vi "Panel.vi"(11 "LightsPanel in":refnum<class "LightsPanel.lvclass">) -> ()   [LabVIEW 2022 SP3, in "TouchControl.lvlib" / "LightsPanel.lvclass"]
uses:
  LightsPanel.lvclass
  C:/Program Files (x86)/National Instruments/LabVIEW 2022/vi.lib/IlluminatedG/IG OOPanel/OOPanel/Panel/Panel.lvclass
  Temperature Meter.ctl
  <vilib>/IlluminatedG/IG OOPanel/OOPanel/Panel/Basic UI State.ctl
  Light Selection.ctl
  <vilib>/IlluminatedG/IG OOPanel/OOPanel/Panel/Panel.lvclass
  <vilib>/IlluminatedG/IG OOPanel/OOPanel/OOPanel.lvlib
  TouchControl.lvlib
panel:
  in  "Printer On":bool
  in  "Desk Right On":bool
  in  "Desk Left On":bool
  in  "Printer Brightness":i32(slide) caption="Printer" scale=3.0..100.0
  in  "Printer Temp":T1 scale=7000.0..2900.0
  in  "Link":bool=TRUE
  in  "Desk Right Temp":T1 scale=7000.0..2900.0
  in  "Desk Right Brightness":i32(slide) caption="Desk Right" scale=3.0..100.0
  in  "Desk Left Temp":T1 scale=7000.0..2900.0
  in  "Desk Left Brightness":i32(slide) caption="Desk Left" scale=3.0..100.0
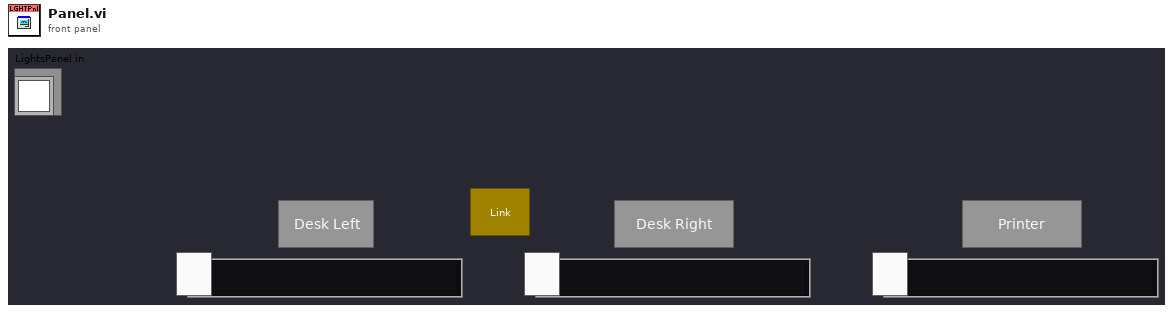
[diagram p1: front panel]
types:
  T1 = typedef "Temperature Meter.ctl" = dbl
  T2 = typedef "OOPanel.lvlib/Panel.lvclass/Basic UI State.ctl" = enum16{"Init", "Run", "Close"}
  T3 = typedef "TouchControl.lvlib/Light Selection.ctl" = enum16{"Desk Left", "Desk Right", "Printer"}
  T4 = typedef "OOPanel.lvlib/Panel.lvclass/Panel Events.ctl" = cluster{"Visbility":refnum<user-event>, "Close":refnum<user-event>}
  T5 = typedef "OOPanel.lvlib/Visibility State.ctl" = enum16{"Idle", "Closed", "Hidden", "Visible", "Subpanel", "Hidden Subpanel"}
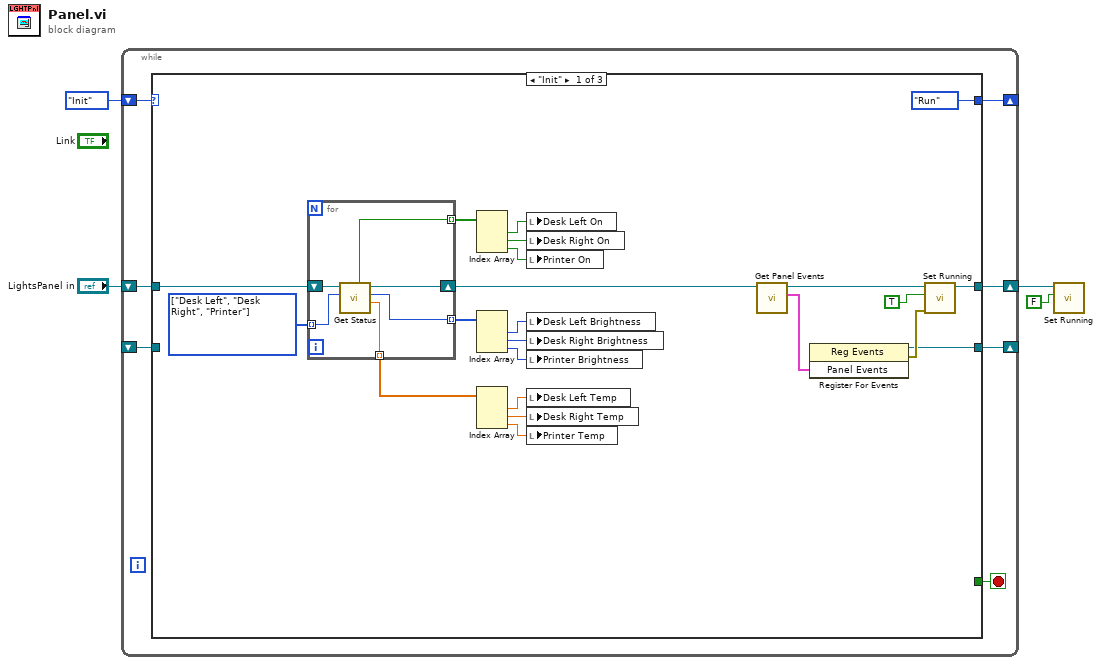
[diagram p0: block diagram]
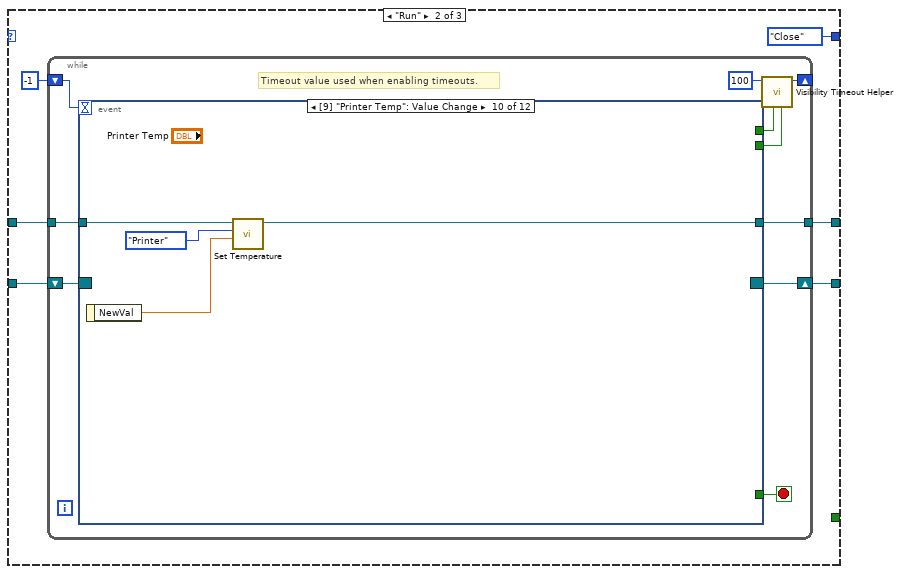
[diagram p2: hidden frame]
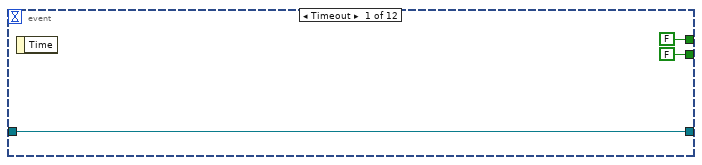
[diagram p3: hidden frame]
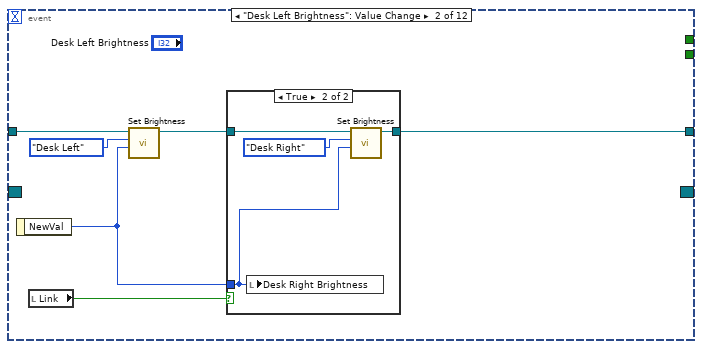
[diagram p4: hidden frame]
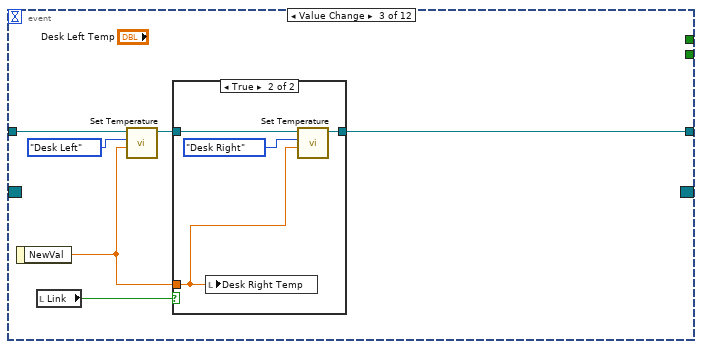
[diagram p6: hidden frame]
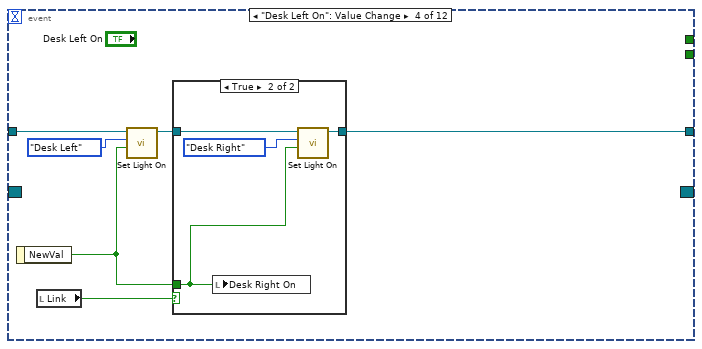
[diagram p8: hidden frame]
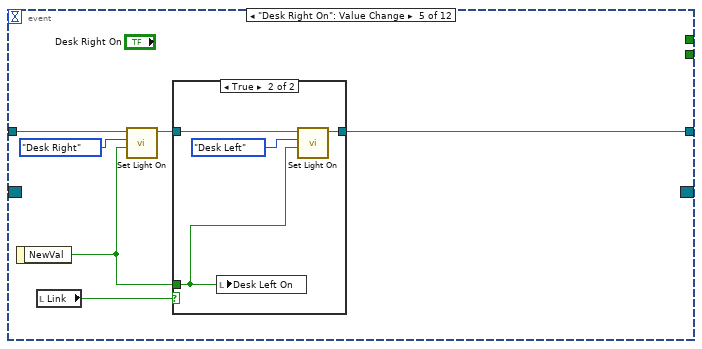
[diagram p10: hidden frame]
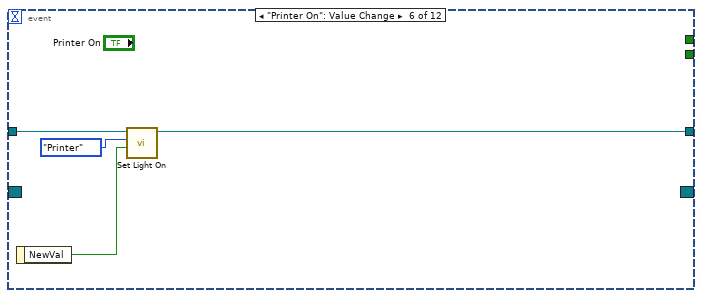
[diagram p12: hidden frame]
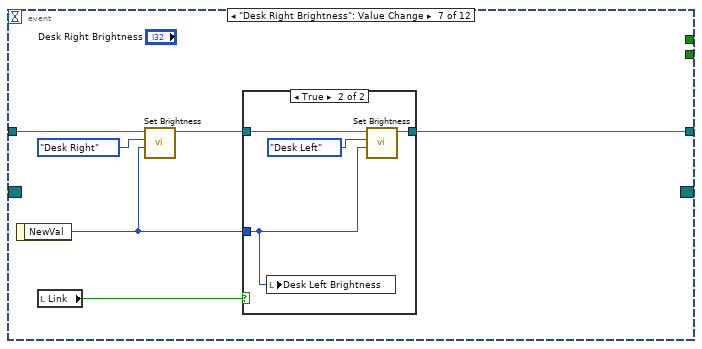
[diagram p13: hidden frame]
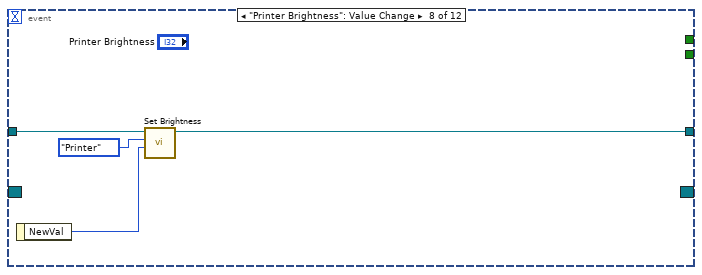
[diagram p15: hidden frame]
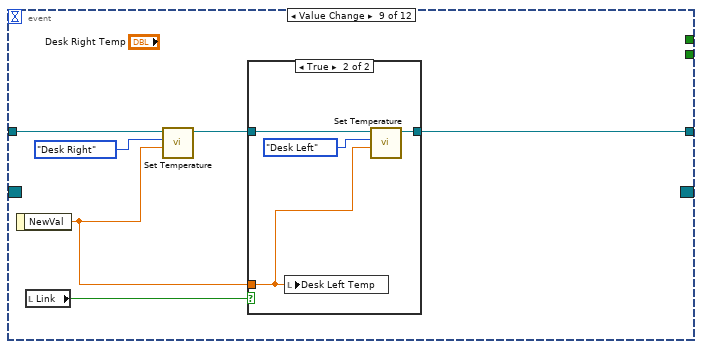
[diagram p16: hidden frame]
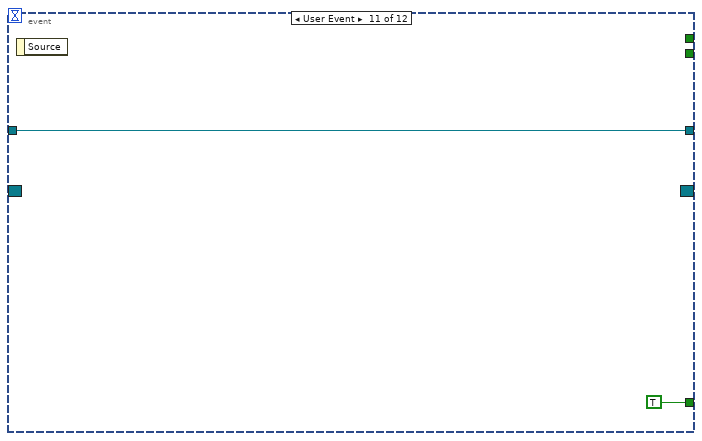
[diagram p18: hidden frame]
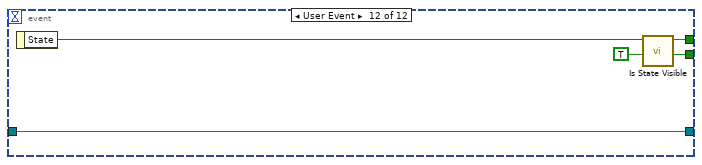
[diagram p19: hidden frame]
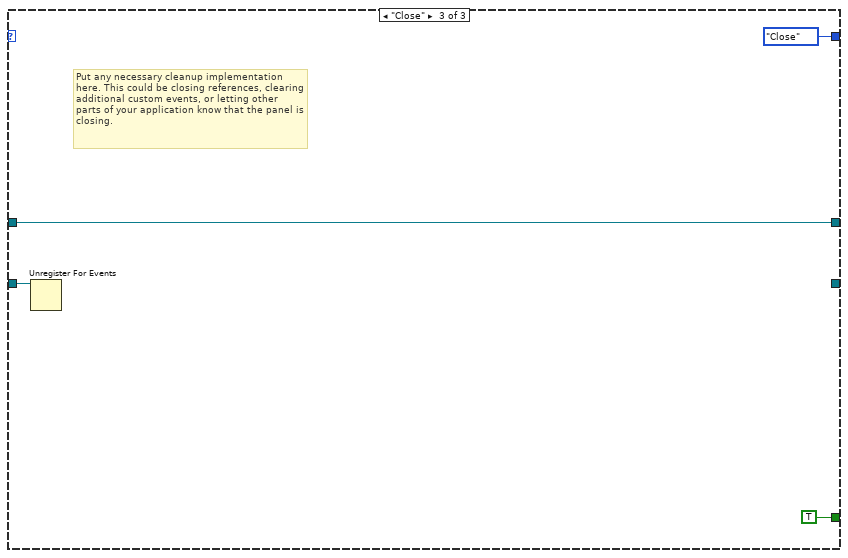
[diagram p20: hidden frame]
diagram:
  n1 = while {
    shift-right: [w10] -> _
    shift-left: _ -> [w11]
    shift-right: [w8] -> _
    shift-left: Basic_UI_State."Init" ("Basic UI State") -> [w9]
    shift-right: [w6] -> w4
    shift-left: "LightsPanel in" -> [w5]
    stop <- w7 stop-if-true
    n2 = case shown="\"Init\"" w9 {
      tunnel: w11 -> [_ w45 w144]
      tunnel: [w30 w43 _] -> w10
      tunnel: [Basic_UI_State."Run" ("Basic UI State") Basic_UI_State."Close" ("Basic UI State") Basic_UI_State."Close" ("Basic UI State")] -> w8
      tunnel: [_ _ TRUE] -> w7
      tunnel: [w29 w40 w143] -> w6
      tunnel: w5 -> [w26 w41 w143]
      frame "Init" {
        w25 = T3[] [enum."Desk Left", enum."Desk Right", enum."Printer"] items=["Desk Left", "Desk Right", "Printer"]
        n3 = for {
          shift-right: [w38] -> w24
          shift-left: w26 -> [w39]
          tunnel: w25 -> [w37] mode=indexing
          tunnel: [w36] -> w23 mode=indexing
          tunnel: [w35] -> w19 mode=indexing
          tunnel: [w34] -> w12 mode=indexing
          n4 = call "Get Status.vi"("Light Selection"=w37, "LightsPanel in"=w39) -> ("Temperature"=w34:dbl, "Brightness"=w35:i32, "LightsPanel out"=w38:refnum<class "LightsPanel.lvclass">, "On"=w36:bool)  [unwired: 5 in, 1 out]
        }
        n5 = Index Array(array=w23) -> (element #1=w20:bool, element #2=w22:bool, element #3=w21:bool)  [unwired: 3 in]
        n6 = Index Array(array=w19) -> (element #1=w17:i32, element #2=w18:i32, element #3=w16:i32)  [unwired: 3 in]
        n7 = Index Array(array=w12) -> (element #1=w14:dbl, element #2=w13:dbl, element #3=w15:dbl)  [unwired: 3 in]
        n8 = local write "Desk Left On"(w20) -> ()
        n9 = local write "Desk Right On"(w22) -> ()
        n10 = local write "Printer On"(w21) -> ()
        n11 = local write "Desk Left Brightness"(w17) -> ()
        n12 = local write "Desk Right Brightness"(w18) -> ()
        n13 = local write "Printer Brightness"(w16) -> ()
        n14 = local write "Desk Left Temp"(w14) -> ()
        n15 = local write "Desk Right Temp"(w13) -> ()
        n16 = local write "Printer Temp"(w15) -> ()
        n17 = call <vilib>:"Get Panel Events.vi"("Panel in"=w24) -> ("Panel Events"=w27:T4, "Panel out"=w28:refnum<class "LightsPanel.lvclass">)  [unwired: 8 in, 1 out]
        n18 = register-events(w27) -> (reference out=w30:refnum<event-registration>, error out=w32:errorcluster)  [unwired: 2 in]
        n19 = call <vilib>:"Set Running.vi"("error in (no error)"=w32, "Running"=TRUE, "Panel in"=w28) -> ("Panel out"=w29:refnum<class "LightsPanel.lvclass">)  [unwired: 7 in, 1 out]
      }
      frame "Run" {
        n20 = while {
          shift-right: [w51] -> w43
          shift-left: w45 -> [w52]
          shift-right: [w54] -> _
          shift-left: -1 ("Timeout") -> [w53]
          tunnel: w41 -> [w47]
          tunnel: [w46] -> w40
          stop <- w48 stop-if-true
          # "Timeout value used when enabling timeouts."
          n21 = event shown="[9] \"Printer Temp\": Value Change" {
            selector: w52 -> [_ _ _ _ _ _ _ _ _ _ _ _]
            dyn-events: [_ _ _ _ _ _ _ _ _ _ _ _] -> w51
            timeout: w53 -> [_ _ _ _ _ _ _ _ _ _ _ _]
            tunnel: [FALSE _ _ _ _ _ _ _ _ _ _ w141] -> w50
            tunnel: [FALSE _ _ _ _ _ _ _ _ _ _ TRUE] -> w49
            tunnel: [_ _ _ _ _ _ _ _ _ _ TRUE _] -> w48
            tunnel: w47 -> [w56 w64 w75 w86 w97 w106 w110 w120 w126 w136 w137 w139]
            tunnel: [w56 w59 w70 w81 w92 w103 w109 w118 w122 w133 w137 w139] -> w46
            event Timeout {
              n22 = event-data() -> ()  [unwired: 1 in, 1 out]
            }
            event "Desk Left Brightness": Value Change {
              n23 = event-data() -> ("NewVal"=w61:i32)  [unwired: 1 in]
              n24 = local read "Link"() -> (w63:bool)
              n25 = call "Set Brightness.vi"("Brightness"=w61, "Light Selection"=Light_Selection."Desk Left", "LightsPanel in"=w64) -> ("LightsPanel out"=w60:refnum<class "LightsPanel.lvclass">)  [unwired: 7 in, 1 out]
              n26 = case shown="True" w63 {
                tunnel: w61 -> [_ w67]
                tunnel: w60 -> [w65 w68]
                tunnel: [w65 w66] -> w59
                frame False {
                }
                frame True {
                  n27 = local write "Desk Right Brightness"(w67) -> ()
                  n28 = call "Set Brightness.vi"("Brightness"=w67, "Light Selection"=Light_Selection."Desk Right", "LightsPanel in"=w68) -> ("LightsPanel out"=w66:refnum<class "LightsPanel.lvclass">)  [unwired: 7 in, 1 out]
                }
              }
            }
            event Value Change {
              n29 = event-data() -> ("NewVal"=w72:T1)  [unwired: 1 in]
              n30 = local read "Link"() -> (w74:bool)
              n31 = call "Set Temperature.vi"("Temperature"=w72, "Light Selection"=Light_Selection."Desk Left", "LightsPanel in"=w75) -> ("LightsPanel out"=w71:refnum<class "LightsPanel.lvclass">)  [unwired: 7 in, 1 out]
              n32 = case shown="True" w74 {
                tunnel: w72 -> [_ w78]
                tunnel: w71 -> [w76 w80]
                tunnel: [w76 w77] -> w70
                frame False {
                }
                frame True {
                  n33 = local write "Desk Right Temp"(w78) -> ()
                  n34 = call "Set Temperature.vi"("Temperature"=w78, "Light Selection"=Light_Selection."Desk Right", "LightsPanel in"=w80) -> ("LightsPanel out"=w77:refnum<class "LightsPanel.lvclass">)  [unwired: 7 in, 1 out]
                }
              }
            }
            event "Desk Left On": Value Change {
              n35 = event-data() -> ("NewVal"=w83:bool)  [unwired: 1 in]
              n36 = local read "Link"() -> (w85:bool)
              n37 = call "Set Light On.vi"("On"=w83, "Light Selection"=Light_Selection."Desk Left", "LightsPanel in"=w86) -> ("LightsPanel out"=w82:refnum<class "LightsPanel.lvclass">)  [unwired: 7 in, 1 out]
              n38 = case shown="True" w85 {
                tunnel: w83 -> [_ w89]
                tunnel: w82 -> [w87 w91]
                tunnel: [w87 w88] -> w81
                frame False {
                }
                frame True {
                  n39 = local write "Desk Right On"(w89) -> ()
                  n40 = call "Set Light On.vi"("On"=w89, "Light Selection"=Light_Selection."Desk Right", "LightsPanel in"=w91) -> ("LightsPanel out"=w88:refnum<class "LightsPanel.lvclass">)  [unwired: 7 in, 1 out]
                }
              }
            }
            event "Desk Right On": Value Change {
              n41 = event-data() -> ("NewVal"=w94:bool)  [unwired: 1 in]
              n42 = local read "Link"() -> (w96:bool)
              n43 = call "Set Light On.vi"("On"=w94, "Light Selection"=Light_Selection."Desk Right", "LightsPanel in"=w97) -> ("LightsPanel out"=w93:refnum<class "LightsPanel.lvclass">)  [unwired: 7 in, 1 out]
              n44 = case shown="True" w96 {
                tunnel: w94 -> [_ w100]
                tunnel: w93 -> [w98 w102]
                tunnel: [w98 w99] -> w92
                frame False {
                }
                frame True {
                  n45 = local write "Desk Left On"(w100) -> ()
                  n46 = call "Set Light On.vi"("On"=w100, "Light Selection"=Light_Selection."Desk Left", "LightsPanel in"=w102) -> ("LightsPanel out"=w99:refnum<class "LightsPanel.lvclass">)  [unwired: 7 in, 1 out]
                }
              }
            }
            event "Printer On": Value Change {
              n47 = event-data() -> ("NewVal"=w104:bool)  [unwired: 1 in]
              n48 = call "Set Light On.vi"("On"=w104, "Light Selection"=Light_Selection."Printer", "LightsPanel in"=w106) -> ("LightsPanel out"=w103:refnum<class "LightsPanel.lvclass">)  [unwired: 7 in, 1 out]
            }
            event "Desk Right Brightness": Value Change {
              n49 = event-data() -> ("NewVal"=w108:i32)  [unwired: 1 in]
              n50 = local read "Link"() -> (w107:bool)
              n51 = call "Set Brightness.vi"("Brightness"=w108, "Light Selection"=Light_Selection."Desk Right", "LightsPanel in"=w110) -> ("LightsPanel out"=w112:refnum<class "LightsPanel.lvclass">)  [unwired: 7 in, 1 out]
              n52 = case shown="True" w107 {
                tunnel: w112 -> [w113 w116]
                tunnel: [w113 w115] -> w109
                tunnel: w108 -> [_ w114]
                frame False {
                }
                frame True {
                  n53 = local write "Desk Left Brightness"(w114) -> ()
                  n54 = call "Set Brightness.vi"("Brightness"=w114, "Light Selection"=Light_Selection."Desk Left", "LightsPanel in"=w116) -> ("LightsPanel out"=w115:refnum<class "LightsPanel.lvclass">)  [unwired: 7 in, 1 out]
                }
              }
            }
            event "Printer Brightness": Value Change {
              n55 = event-data() -> ("NewVal"=w119:i32)  [unwired: 1 in]
              n56 = call "Set Brightness.vi"("Brightness"=w119, "Light Selection"=Light_Selection."Printer", "LightsPanel in"=w120) -> ("LightsPanel out"=w118:refnum<class "LightsPanel.lvclass">)  [unwired: 7 in, 1 out]
            }
            event Value Change {
              n57 = event-data() -> ("NewVal"=w124:T1)  [unwired: 1 in]
              n58 = local read "Link"() -> (w127:bool)
              n59 = call "Set Temperature.vi"("Temperature"=w124, "Light Selection"=Light_Selection."Desk Right", "LightsPanel in"=w126) -> ("LightsPanel out"=w123:refnum<class "LightsPanel.lvclass">)  [unwired: 7 in, 1 out]
              n60 = case shown="True" w127 {
                tunnel: w124 -> [_ w130]
                tunnel: w123 -> [w128 w132]
                tunnel: [w128 w129] -> w122
                frame False {
                }
                frame True {
                  n61 = local write "Desk Left Temp"(w130) -> ()
                  n62 = call "Set Temperature.vi"("Temperature"=w130, "Light Selection"=Light_Selection."Desk Left", "LightsPanel in"=w132) -> ("LightsPanel out"=w129:refnum<class "LightsPanel.lvclass">)  [unwired: 7 in, 1 out]
                }
              }
            }
            event Value Change {
              n63 = event-data() -> ("NewVal"=w134:T1)  [unwired: 1 in]
              n64 = call "Set Temperature.vi"("Temperature"=w134, "Light Selection"=Light_Selection."Printer", "LightsPanel in"=w136) -> ("LightsPanel out"=w133:refnum<class "LightsPanel.lvclass">)  [unwired: 7 in, 1 out]
            }
            event User Event {
              n65 = event-data() -> ()  [unwired: 1 in, 1 out]
            }
            event User Event {
              n66 = event-data() -> ("State"=w142:T5)  [unwired: 1 in]
              n67 = call <vilib>:"Is State Visible.vi"("Visibility"=w142) -> ("Visible"=w141:bool)  [unwired: 10 in]
            }
          }
          n68 = call <vilib>:"Visibility Timeout Helper.vi"("Update?"=w49, "Use Timeout?"=w50, "Visible Timeout mS"=100) -> ("Timeout"=w54:i32)  [unwired: 8 in]
        }
      }
      frame "Close" {
        # "Put any necessary cleanup implementation here. This could be closing references, clearing additional custom events, or letting other parts of your application know that the panel is closing."
        n69 = Unregister For Events(event registration refnum=w144) -> ()  [unwired: 1 in, 1 out]
      }
    }
  }
  n70 = call <vilib>:"Set Running.vi"("Running"=FALSE, "Panel in"=w4) -> ()  [unwired: 8 in, 2 out]
